vi "Validate_Init.vi"(0 "scripts manager in":refnum<class "scripts manager.lvclass">, 11 "error in (no error)":errorcluster) -> (4 "scripts manager out":refnum<class "scripts manager.lvclass">, 15 "error out":errorcluster)   [LabVIEW 2019, in "LSL.lvlib" / "scripts manager.lvclass"]
uses:
  scripts manager.lvclass
  functions/functionsbase/functionbase.lvclass
  common/line and indent/Line Details.ctl
  scripts manager.lvclass/scripts manager.ctl
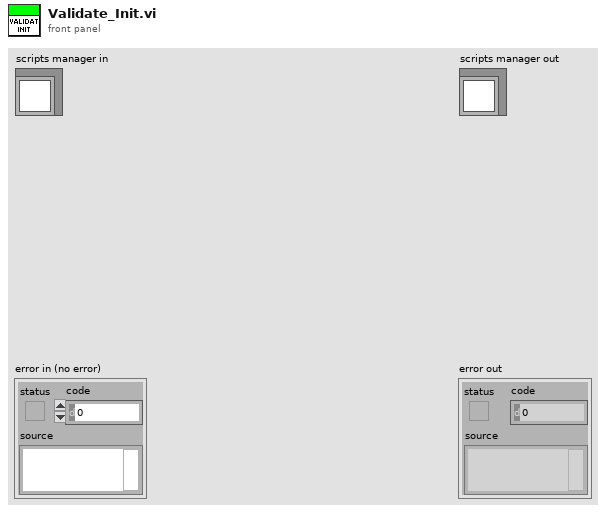
[diagram p1: front panel]
types:
  T1 = typedef "Line Details.ctl" = cluster{"Line#":i64, "Indent#":i64, "Function":string}
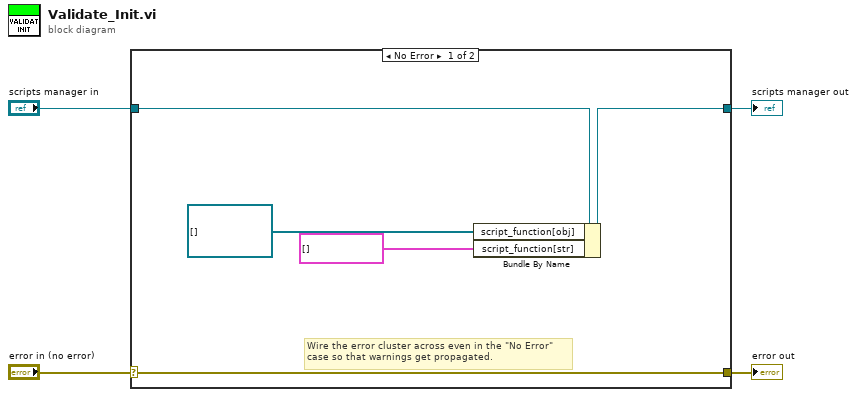
[diagram p0: block diagram]
diagram:
  n1 = case shown="No Error" "error in (no error)" {
    selector: "error in (no error)" -> [w9 w11]
    tunnel: [w9 w11] -> w3
    tunnel: [w7 w10] -> w1
    tunnel: "scripts manager in" -> [w8 w10]
    frame No Error {
      # "Wire the error cluster across even in the \"No Error\"\ncase so that warnings get propagated."
      n2 = Bundle By Name(cluster=w8, "script_function[obj]"=refnum<class "functionbase.lvclass">[] [], "script_function[str]"=T1[] []) -> (w7:refnum<class "scripts manager.lvclass">)
    }
    frame Error {
    }
  }
  "error out" <- w3
  "scripts manager out" <- w1
